vi "从数据库获取数据通用可配置(子VI).vi"(8 "错误输入（无错误）":errorcluster, 9 "查询参数数组":string[](array[string])=["CODMn", "CODCr", "DO", "DOper", "PH", "氨氮", "比电导率", "水温", "盐度", "浊度", "总氮", "总磷", "叶绿素", "藻密度"], 10 "table输入":string="实时数据", 11 "列队名（唯一）":string) -> (0 "错误输出":errorcluster, 3 "簇数组":cluster{"待发送数据":string[][]}[][](array[cluster]))   [LabVIEW 2016, in "数据传输系统.lvlib"]
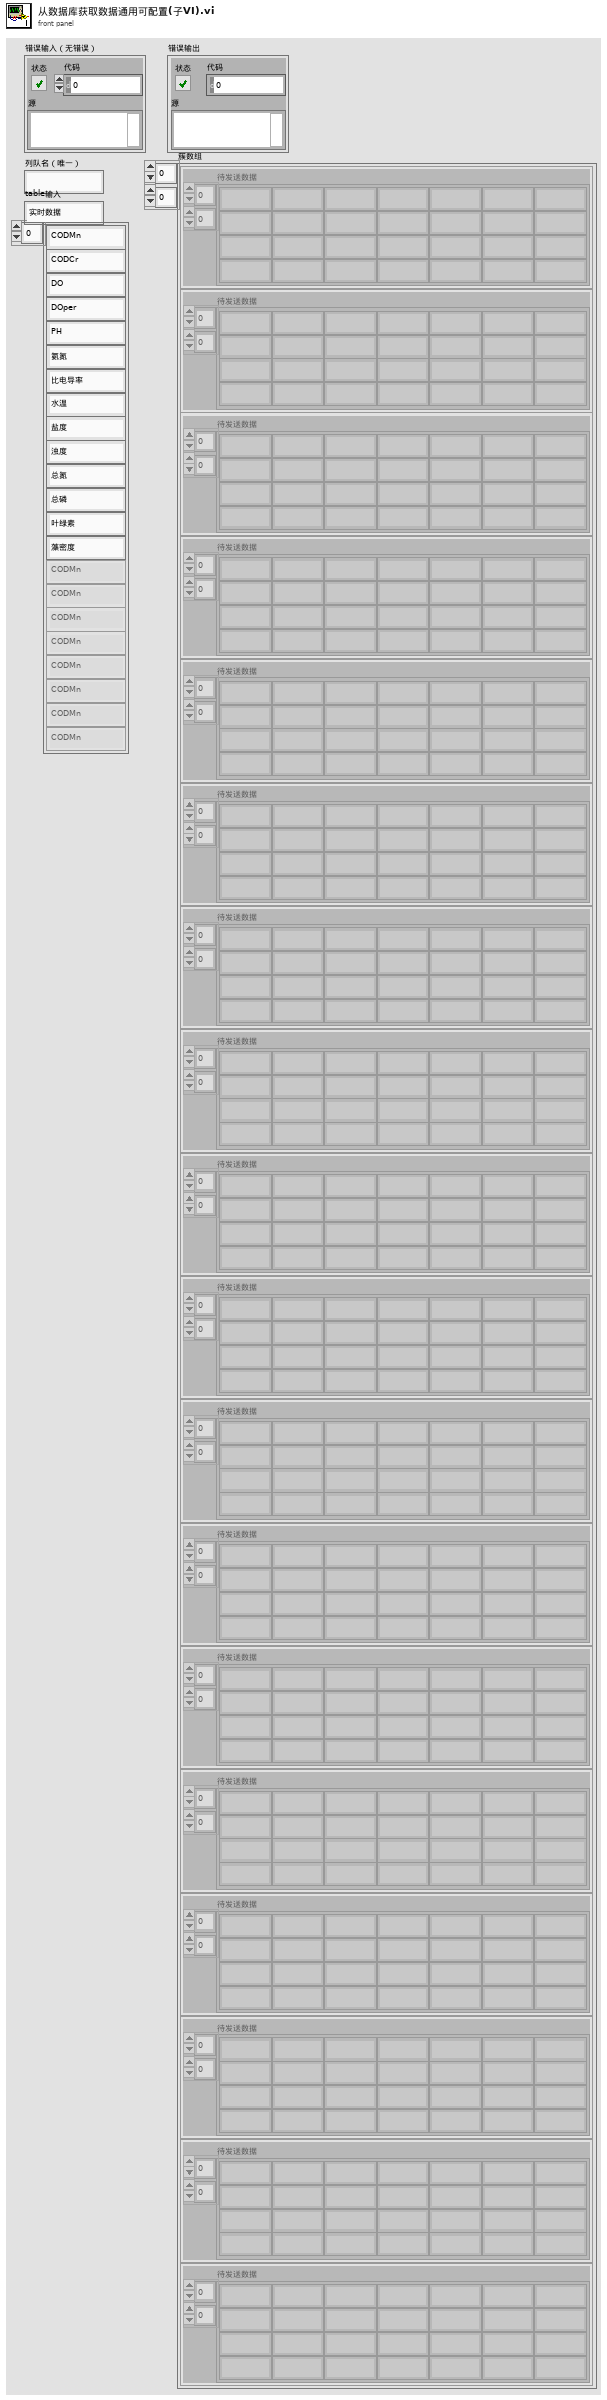
[diagram p1: front panel]
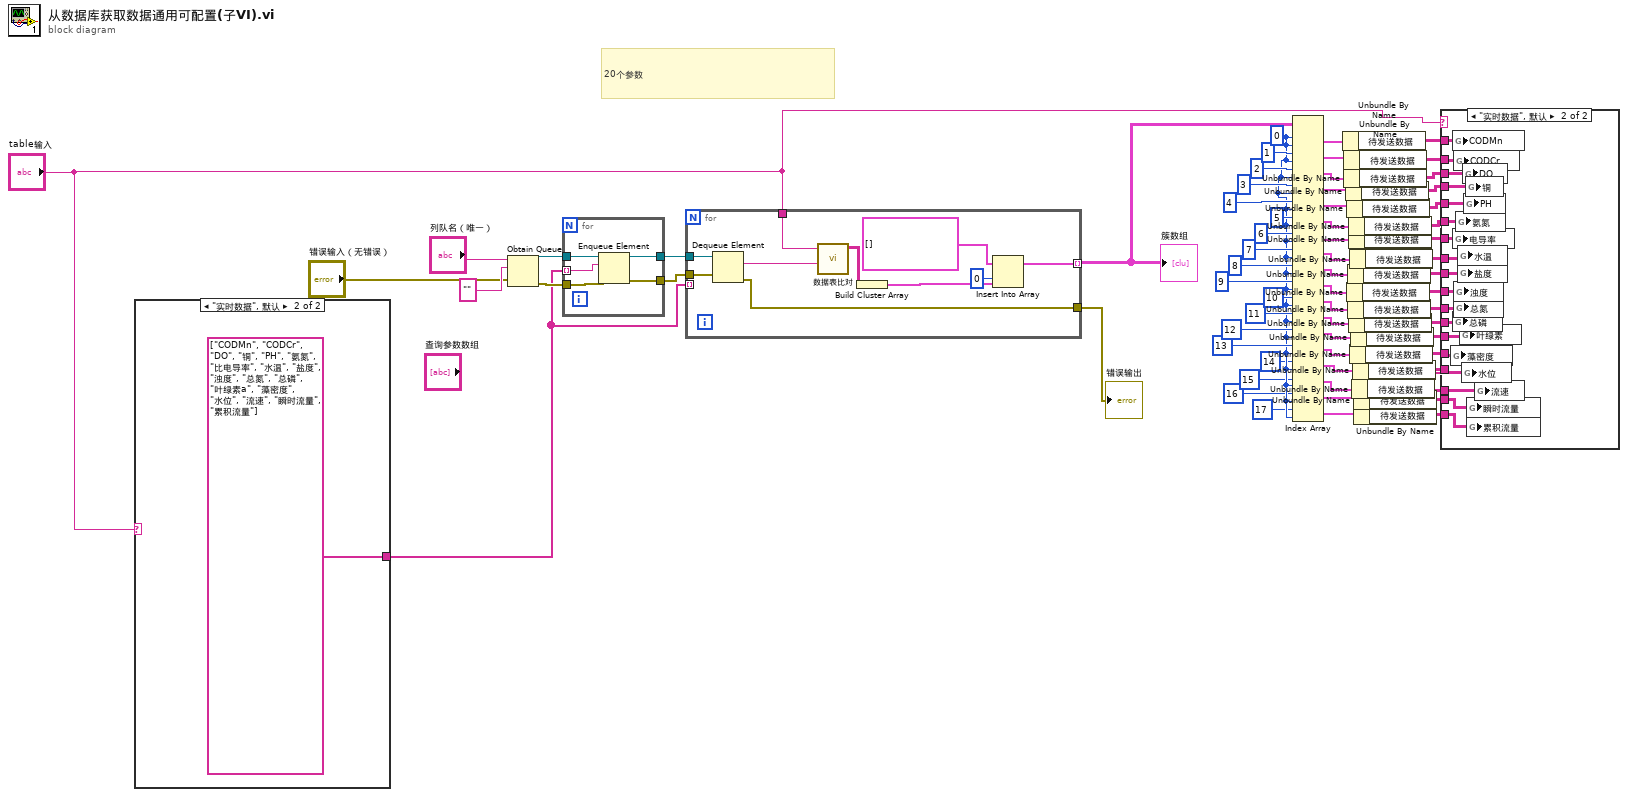
[diagram p0: block diagram]
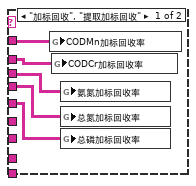
[diagram p2: hidden frame]
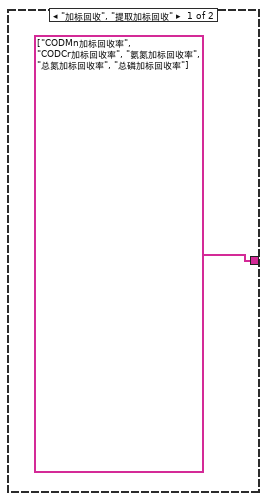
[diagram p3: hidden frame]
diagram:
  w14 = 0 ("索引 (行)")
  # "20个参数"
  n1 = case shown="\"实时数据\", 默认" "table输入" {
    tunnel: [string[] ["CODMn加标回收率", "CODCr加标回收率", "氨氮加标回收率", "总氮加标回收率", "总磷加标回收率"] ("查询参数数组") string[] ["CODMn", "CODCr", "DO", "铜", "PH", "氨氮", "比电导率", "水温", "盐度", "浊度", "总氮", "总磷", "叶绿素a", "藻密度", "水位", "流速", "瞬时流量", "累积流量"] ("查询参数数组")] -> w15
    frame "加标回收", "提取加标回收" {
    }
    frame "实时数据", Default {
    }
  }
  n2 = Obtain Queue(name (unnamed)="列队名（唯一）", element data type="" ("名称（未命名）"), error in (no error)="错误输入（无错误）") -> (queue out=w63:refnum<queue>, error out=w62:errorcluster)  [unwired: 2 in, 1 out]
  n3 = for {
    tunnel: w15 -> [w70] mode=indexing
    tunnel: w63 -> [w72]
    tunnel: w62 -> [w71]
    tunnel: [w69] -> w61
    tunnel: [w68] -> w60
    n4 = Enqueue Element(queue=w72, element=w70, error in (no error)=w71) -> (queue out=w69:refnum<queue>, error out=w68:errorcluster)  [unwired: 1 in, 1 out]
  }
  n5 = for {
    tunnel: w15 -> [_] mode=indexing
    tunnel: w61 -> [w82]
    tunnel: w60 -> [w81]
    tunnel: [w77] -> w57 mode=indexing
    tunnel: "table输入" -> [w74]
    tunnel: [w73] -> w58
    n6 = Dequeue Element(queue=w82, error in (no error)=w81) -> (element=w80:string, error out=w73:errorcluster)  [unwired: 1 in, 2 out]
    n7 = call "数据表比对.vi"("查询元素输入"=w80, "table输入"=w74) -> ("待发送数据"=w79:string[][])  [unwired: 6 in, 3 out]
    n8 = Build Cluster Array(w79) -> (w78:cluster{"待发送数据":string[][]}[])
    n9 = Insert Into Array(array=cluster{"待发送数据":string[][]}[] [] ("簇数组"), index=0 ("索引"), new element=w78) -> (w77:cluster{"待发送数据":string[][]}[])
  }
  "簇数组" <- w57
  "错误输出" <- w58
  n10 = Index Array(array=w57, index (row) #1=w14, index (col) #1=w14, index (row) #2=1 ("索引 (行)"), index (col) #2=w14, index (row) #3=2 ("索引 (行)"), index (col) #3=w14, index (row) #4=3 ("索引 (行)"), index (col) #4=w14, index (row) #5=4 ("索引 (行)"), index (col) #5=w14, index (row) #6=5 ("索引 (行)"), index (col) #6=w14, index (row) #7=6 ("索引 (行)"), index (col) #7=w14, index (row) #8=7 ("索引 (行)"), index (col) #8=w14, index (row) #9=8 ("索引 (行)"), index (col) #9=w14, index (row) #10=9 ("索引 (行)"), index (col) #10=w14, index (row) #11=10 ("索引 (行)"), index (col) #11=w14, index (row) #12=11 ("索引 (行)"), index (col) #12=w14, index (row) #13=12 ("索引 (行)"), index (col) #13=w14, index (row) #14=13 ("索引 (行)"), index (col) #14=w14, index (row) #15=14 ("禁用的索引 (行)"), index (col) #15=w14, index (row) #16=15 ("禁用的索引 (行)"), index (col) #16=w14, index (row) #17=16 ("禁用的索引 (行)"), index (col) #17=w14, index (row) #18=17 ("禁用的索引 (行)"), index (col) #18=w14) -> (element #1=w56:cluster{"待发送数据":string[][]}, element #2=w41:cluster{"待发送数据":string[][]}, element #3=w40:cluster{"待发送数据":string[][]}, element #4=w39:cluster{"待发送数据":string[][]}, element #5=w38:cluster{"待发送数据":string[][]}, element #6=w37:cluster{"待发送数据":string[][]}, element #7=w35:cluster{"待发送数据":string[][]}, element #8=w36:cluster{"待发送数据":string[][]}, element #9=w34:cluster{"待发送数据":string[][]}, element #10=w33:cluster{"待发送数据":string[][]}, element #11=w32:cluster{"待发送数据":string[][]}, element #12=w31:cluster{"待发送数据":string[][]}, element #13=w30:cluster{"待发送数据":string[][]}, element #14=w29:cluster{"待发送数据":string[][]}, element #15=w9:cluster{"待发送数据":string[][]}, element #16=w7:cluster{"待发送数据":string[][]}, element #17=w6:cluster{"待发送数据":string[][]}, element #18=w5:cluster{"待发送数据":string[][]})
  n11 = Unbundle By Name(w56) -> ("待发送数据"=w55:string[][])
  n12 = Unbundle By Name(w41) -> ("待发送数据"=w28:string[][])
  n13 = Unbundle By Name(w40) -> ("待发送数据"=w27:string[][])
  n14 = Unbundle By Name(w39) -> ("待发送数据"=w26:string[][])
  n15 = Unbundle By Name(w38) -> ("待发送数据"=w25:string[][])
  n16 = Unbundle By Name(w33) -> ("待发送数据"=w20:string[][])
  n17 = Unbundle By Name(w34) -> ("待发送数据"=w21:string[][])
  n18 = Unbundle By Name(w32) -> ("待发送数据"=w19:string[][])
  n19 = Unbundle By Name(w37) -> ("待发送数据"=w24:string[][])
  n20 = Unbundle By Name(w35) -> ("待发送数据"=w23:string[][])
  n21 = Unbundle By Name(w31) -> ("待发送数据"=w18:string[][])
  n22 = Unbundle By Name(w36) -> ("待发送数据"=w22:string[][])
  n23 = Unbundle By Name(w29) -> ("待发送数据"=w17:string[][])
  n24 = Unbundle By Name(w30) -> ("待发送数据"=w16:string[][])
  n25 = Unbundle By Name(w7) -> ("待发送数据"=w4:string[][])
  n26 = Unbundle By Name(w9) -> ("待发送数据"=w8:string[][])
  n27 = Unbundle By Name(w6) -> ("待发送数据"=w3:string[][])
  n28 = Unbundle By Name(w5) -> ("待发送数据"=w2:string[][])
  n29 = case shown="\"实时数据\", 默认" "table输入" {
    tunnel: w55 -> [w87 w105]
    tunnel: w28 -> [w86 w104]
    tunnel: w27 -> [w85 w103]
    tunnel: w26 -> [w84 w102]
    tunnel: w25 -> [w83 w101]
    tunnel: w24 -> [_ w100]
    tunnel: w23 -> [_ w99]
    tunnel: w22 -> [_ w98]
    tunnel: w21 -> [_ w97]
    tunnel: w20 -> [_ w96]
    tunnel: w19 -> [_ w95]
    tunnel: w18 -> [_ w94]
    tunnel: w17 -> [_ w93]
    tunnel: w16 -> [_ w92]
    tunnel: w8 -> [_ w91]
    tunnel: w4 -> [_ w90]
    tunnel: w3 -> [_ w89]
    tunnel: w2 -> [_ w88]
    frame "加标回收", "提取加标回收" {
      n30 = global write "全局 所有参数.vi" "CODMn加标回收率"(w87) -> ()
      n31 = global write "全局 所有参数.vi" "CODCr加标回收率"(w86) -> ()
      n32 = global write "全局 所有参数.vi" "氨氮加标回收率"(w85) -> ()
      n33 = global write "全局 所有参数.vi" "总氮加标回收率"(w84) -> ()
      n34 = global write "全局 所有参数.vi" "总磷加标回收率"(w83) -> ()
    }
    frame "实时数据", Default {
      n35 = global write "全局 所有参数.vi" "藻密度"(w93) -> ()
      n36 = global write "全局 所有参数.vi" "CODMn"(w105) -> ()
      n37 = global write "全局 所有参数.vi" "电导率"(w99) -> ()
      n38 = global write "全局 所有参数.vi" "总磷"(w94) -> ()
      n39 = global write "全局 所有参数.vi" "CODCr"(w104) -> ()
      n40 = global write "全局 所有参数.vi" "浊度"(w96) -> ()
      n41 = global write "全局 所有参数.vi" "总氮"(w95) -> ()
      n42 = global write "全局 所有参数.vi" "氨氮"(w100) -> ()
      n43 = global write "全局 所有参数.vi" "水温"(w98) -> ()
      n44 = global write "全局 所有参数.vi" "盐度"(w97) -> ()
      n45 = global write "全局 所有参数.vi" "叶绿素"(w92) -> ()
      n46 = global write "全局 所有参数.vi" "水位"(w91) -> ()
      n47 = global write "全局 所有参数.vi" "DO"(w103) -> ()
      n48 = global write "全局 所有参数.vi" "PH"(w101) -> ()
      n49 = global write "全局 所有参数.vi" "铜"(w102) -> ()
      n50 = global write "全局 所有参数.vi" "瞬时流量"(w89) -> ()
      n51 = global write "全局 所有参数.vi" "累积流量"(w88) -> ()
      n52 = global write "全局 所有参数.vi" "流速"(w90) -> ()
    }
  }
